vi "GUI_Bella_FilterWheels_All.vi"() -> ()   [LabVIEW 2013]
uses:
  shared programs/GUI_Template/GUI_master/tcp_new_data_event.ctl
  shared programs/GUI_Template/GUI_master/tcp new data cluster.ctl
panel:
  in  "GUIdevice 4":string="BELLA_ESP_2"
  in  "GUIdevice 3":string="BELLA_ESP_2"
  in  "GUIdevice 2":string="BELLA_ESP_2"
  in  "GUIdevice 1":string="BELLA_ESP_2"
  out "tcp data event":T1
  in  "stop":bool
  out "error IO 2":errorcluster
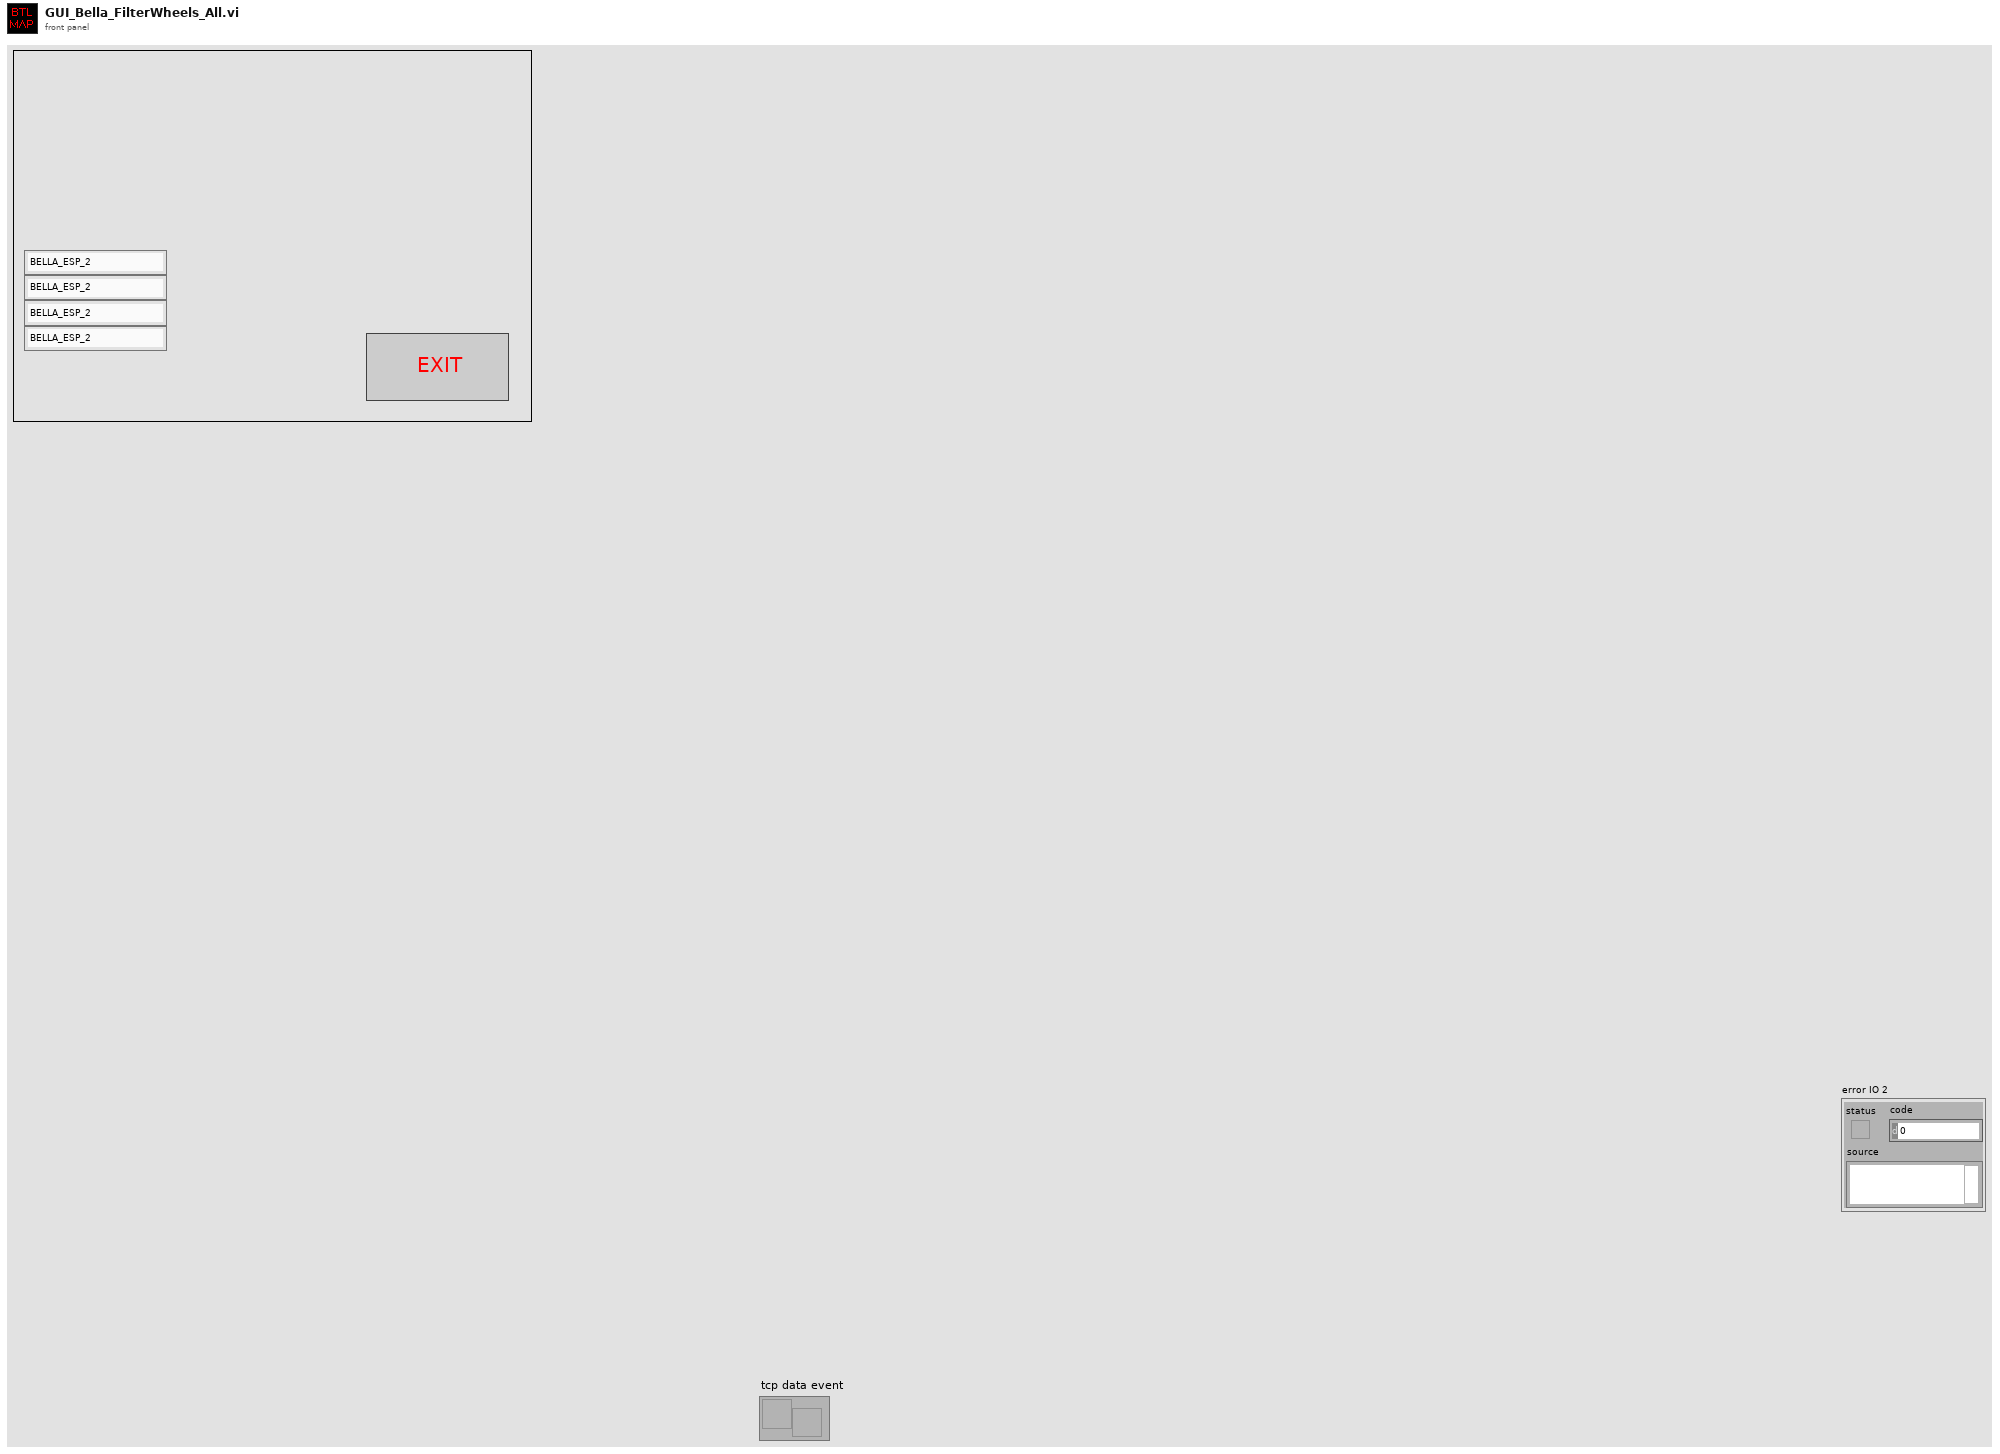
[diagram p1: front panel]
types:
  T1 = typedef "tcp_new_data_event.ctl" = refnum<user-event>
  T2 = typedef "tcp new data cluster.ctl" = cluster{"EventEnum":enum16{"new data", "connection status update"}, "Device name":string}
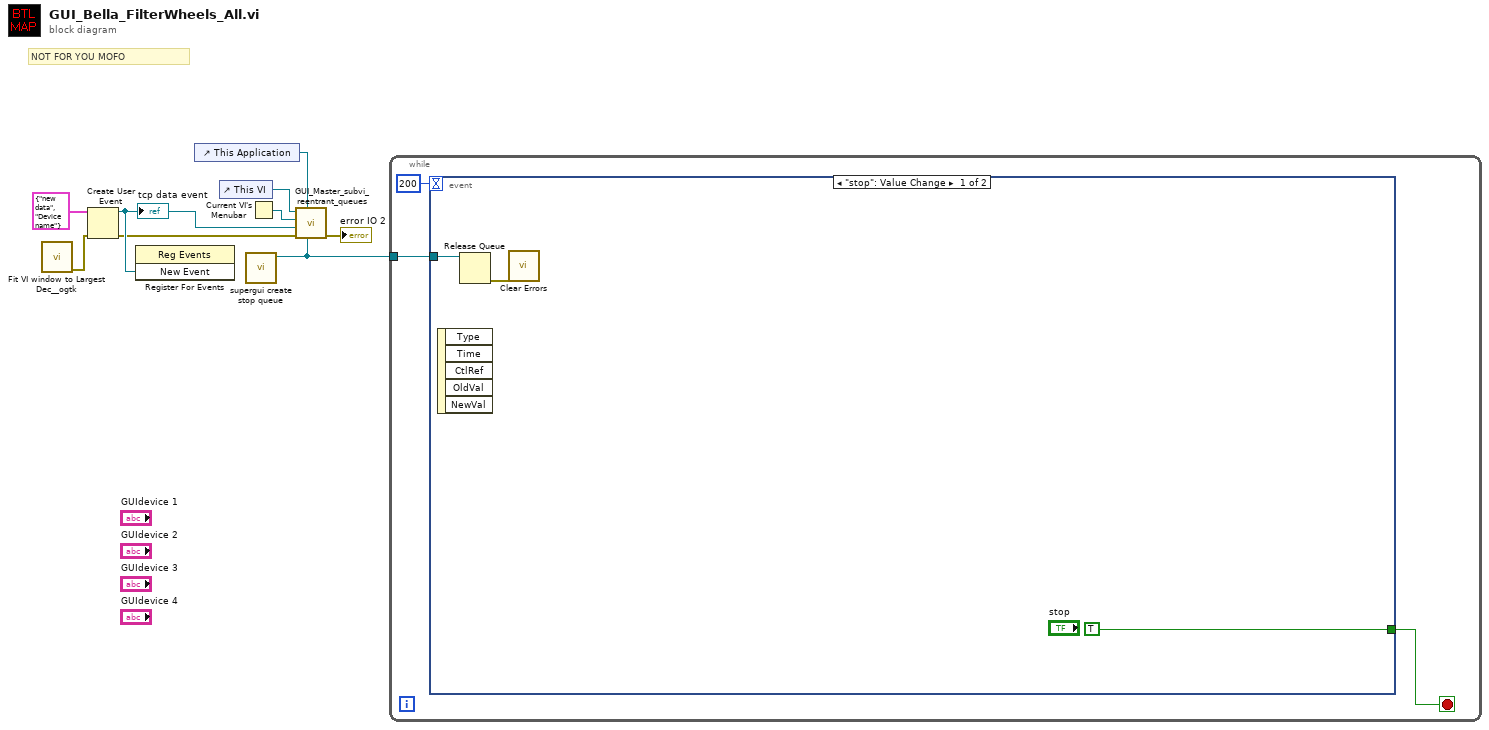
[diagram p0: block diagram]
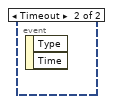
[diagram p2: hidden frame]
diagram:
  # "NOT FOR YOU MOFO"
  n1 = call <userlib>:"Fit VI window to Largest Dec__ogtk.vi"() -> ("error out"=w1:errorcluster)  [unwired: 6 in, 1 out]
  n2 = Create User Event(user event datatype=T2 {"EventEnum"=enum."new data", "Device name"="Device name"} ("New Event"), error in=w1) -> (user event=w8:refnum<user-event>, error out=w7:errorcluster)
  "tcp data event" <- w8
  n3 = register-events(w8) -> ()  [unwired: 2 in, 2 out]
  n4 = control-ref of="This Application"() -> (w9:refnum<vi>)
  n5 = control-ref of="This VI"() -> (w4:refnum<vi>)
  n6 = call "supergui create stop queue.vi"() -> ("STOP Queue out"=w2:refnum<queue>)  [unwired: 11 in]
  n7 = Current VI's Menubar() -> (w5:refnum<k9>)
  n8 = call "GUI_Master_subvi_reentrant_queues.vi"("STOP Queue in"=w2, "This Application"=w9, "error in (no error)"=w7, "tcp data event"=w8, "Caller menu reference"=w5, "Caller VI ref"=w4) -> ("error out"=→"error IO 2":errorcluster)  [unwired: 5 in]
  n9 = while {
    tunnel: w2 -> [w10]
    stop <- w12 stop-if-true
    n10 = event shown="[0] \"stop\": Value Change" {
      selector: _ -> [_ _]
      dyn-events: _ -> [_ _]
      timeout: 200 -> [_ _]
      tunnel: [TRUE ("stop") _] -> w12
      tunnel: w10 -> [w13 _]
      event "stop": Value Change {
        n11 = event-data() -> ()  [unwired: 1 in, 5 out]
        n12 = Release Queue(queue=w13) -> (error out=w14:errorcluster)  [unwired: 2 in, 2 out]
        n13 = call <vilib>:"Clear Errors.vi"("error in (no error)"=w14) -> ()  [unwired: 6 in, 1 out]
      }
      event Timeout {
        n14 = event-data() -> ()  [unwired: 1 in, 2 out]
      }
    }
  }
